vi "Graf.vi"(9 "mód":enum16{"három", "összes", "eleje", "vége"}(ring), 11 "F_kulso_vektor":dbl[][](array[numeric])) -> (3 "Grafikonra":dbl[][](array[numeric]))   [LabVIEW 2013]
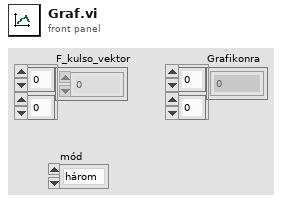
[diagram p1: front panel]
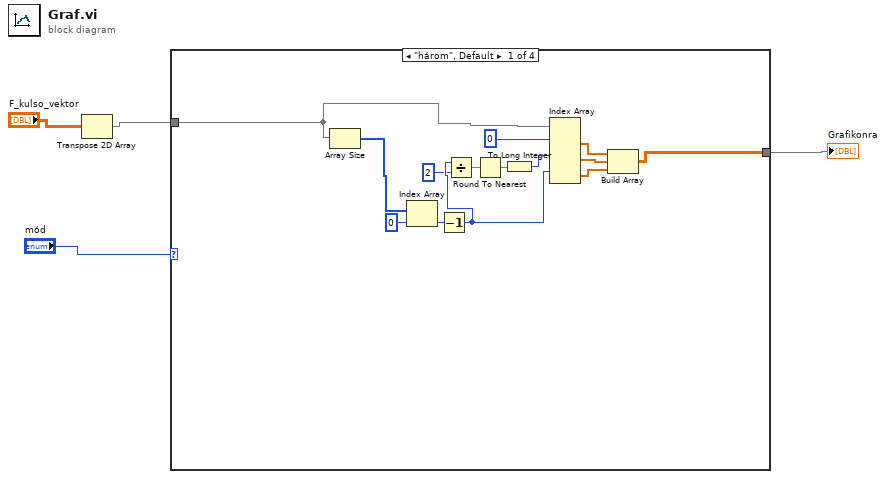
[diagram p0: block diagram]
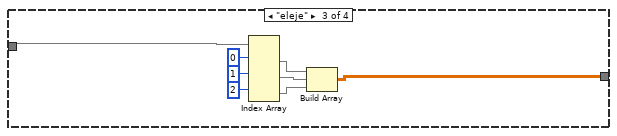
[diagram p3: hidden frame]
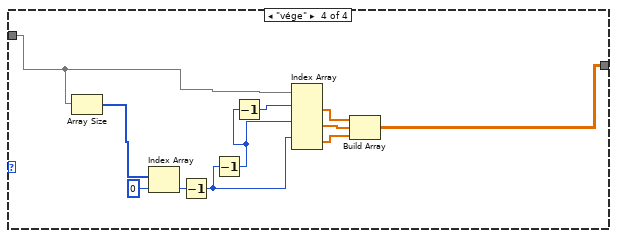
[diagram p4: hidden frame]
diagram:
  n1 = Transpose 2D Array(2D array="F_kulso_vektor") -> (transposed array=w1:dbl[][])
  n2 = case shown="\"három\", Default" "mód" {
    tunnel: w1 -> [w11 w19 w20 w34]
    tunnel: [w12 w19 w21 w35] -> w3
    frame "három", Default {
      n3 = Array Size(array=w11) -> (size(s)=w15:i32[])
      n4 = Index Array(array=w15, index=0) -> (element=w13:i32)
      n5 = Decrement(x=w13) -> (x-1=w8:i32)
      n6 = Divide(x=w8, y=2) -> (x/y=w9:dbl)
      n7 = Round To Nearest(number=w9) -> (nearest integer value=w6:dbl)
      n8 = To Long Integer(number=w6) -> (32bit integer=w5:i32)
      n9 = Index Array(array=w11, index (row) #1=0 ("index (row)"), index (row) #2=w5, index (row) #3=w8) -> (element #1=w16:dbl[], element #2=w17:dbl[], element #3=w18:dbl[])  [unwired: 3 in]
      n10 = Build Array(w16, w17, w18) -> (w12:dbl[][])
    }
    frame "összes" {
    }
    frame "eleje" {
      n11 = Index Array(array=w20, index (row) #1=0 ("index (row)"), index (row) #2=1 ("index (row)"), index (row) #3=2 ("index (row)")) -> (element #1=w25:dbl[], element #2=w24:dbl[], element #3=w22:dbl[])  [unwired: 3 in]
      n12 = Build Array(w25, w24, w22) -> (w21:dbl[][])
    }
    frame "vége" {
      n13 = Array Size(array=w34) -> (size(s)=w33:i32[])
      n14 = Index Array(array=w33, index=0) -> (element=w31:i32)
      n15 = Decrement(x=w31) -> (x-1=w30:i32)
      n16 = Decrement(x=w30) -> (x-1=w28:i32)
      n17 = Decrement(x=w28) -> (x-1=w29:i32)
      n18 = Index Array(array=w34, index (row) #1=w29, index (row) #2=w28, index (row) #3=w30) -> (element #1=w36:dbl[], element #2=w37:dbl[], element #3=w38:dbl[])  [unwired: 3 in]
      n19 = Build Array(w36, w37, w38) -> (w35:dbl[][])
    }
  }
  "Grafikonra" <- w3
